vi "CLD 17 GUI number pad.vi"() -> ()   [LabVIEW 2015]
doc: "CLD 17\n\nThis VI uses a polling method to respond to changes in the GUI."
uses:
  CLD 17 Keypad_Typedef.ctl
panel:
  out "String":string="0"
  out "Numeric":dbl
  in  "Keypad Cluster":T1
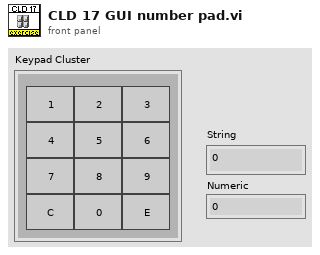
[diagram p1: front panel]
types:
  T1 = typedef "CLD 17 Keypad_Typedef.ctl" = cluster{"0":bool, "1":bool, "2":bool, "3":bool, "4":bool, "5":bool, "6":bool, "7":bool, "8":bool, "9":bool, "C":bool, "E":bool}
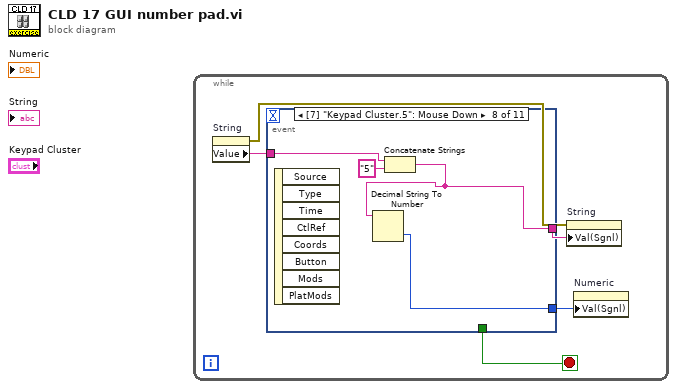
[diagram p0: block diagram]
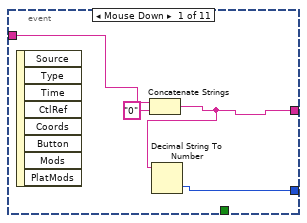
[diagram p2: hidden frame]
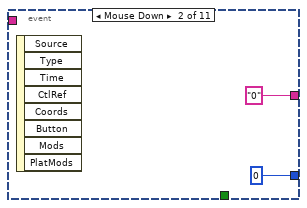
[diagram p3: hidden frame]
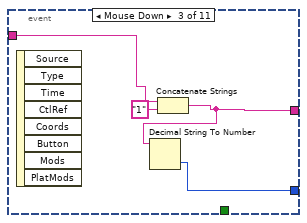
[diagram p4: hidden frame]
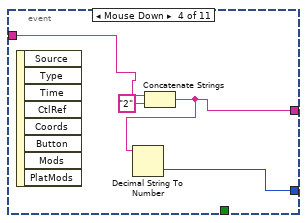
[diagram p5: hidden frame]
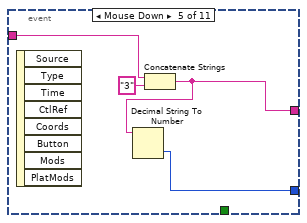
[diagram p6: hidden frame]
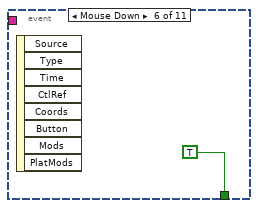
[diagram p7: hidden frame]
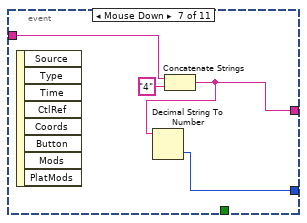
[diagram p8: hidden frame]
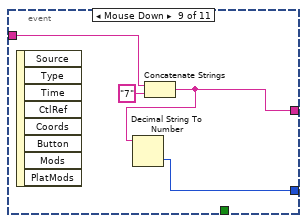
[diagram p9: hidden frame]
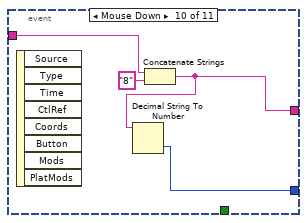
[diagram p10: hidden frame]
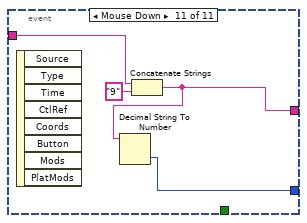
[diagram p11: hidden frame]
diagram:
  n1 = while {
    stop <- w5 stop-if-true
    n2 = property on="String" class="Str"() -> (error out=w2:errorcluster, "Value"=w4:string)  [unwired: 2 in, 1 out]
    n3 = event shown="[7] \"Keypad Cluster.5\": Mouse Down" {
      selector: _ -> [_ _ _ _ _ _ _ _ _ _ _]
      dyn-events: _ -> [_ _ _ _ _ _ _ _ _ _ _]
      timeout: _ -> [_ _ _ _ _ _ _ _ _ _ _]
      tunnel: [_ _ _ _ _ TRUE _ _ _ _ _] -> w5
      tunnel: w4 -> [w8 _ w14 w18 w22 _ w27 w30 w34 w37 w43]
      tunnel: [w6 "0" w12 w16 w21 _ w26 w31 w36 w39 w42] -> w3
      tunnel: [w7 0 w13 w17 w20 _ w25 w29 w33 w38 w41] -> w1
      event Mouse Down {
        n4 = event-data() -> ()  [unwired: 1 in, 8 out]
        n5 = Concatenate Strings(w8, "0" ("string")) -> (w6:string)
        n6 = Decimal String To Number(string=w6) -> (number=w7:i32)  [unwired: 2 in, 1 out]
      }
      event Mouse Down {
        n7 = event-data() -> ()  [unwired: 1 in, 8 out]
      }
      event Mouse Down {
        n8 = event-data() -> ()  [unwired: 1 in, 8 out]
        n9 = Concatenate Strings(w14, "1" ("string")) -> (w12:string)
        n10 = Decimal String To Number(string=w12) -> (number=w13:i32)  [unwired: 2 in, 1 out]
      }
      event Mouse Down {
        n11 = event-data() -> ()  [unwired: 1 in, 8 out]
        n12 = Concatenate Strings(w18, "2" ("string")) -> (w16:string)
        n13 = Decimal String To Number(string=w16) -> (number=w17:i32)  [unwired: 2 in, 1 out]
      }
      event Mouse Down {
        n14 = event-data() -> ()  [unwired: 1 in, 8 out]
        n15 = Concatenate Strings(w22, "3" ("string")) -> (w21:string)
        n16 = Decimal String To Number(string=w21) -> (number=w20:i32)  [unwired: 2 in, 1 out]
      }
      event Mouse Down {
        n17 = event-data() -> ()  [unwired: 1 in, 8 out]
      }
      event Mouse Down {
        n18 = event-data() -> ()  [unwired: 1 in, 8 out]
        n19 = Concatenate Strings(w27, "4" ("string")) -> (w26:string)
        n20 = Decimal String To Number(string=w26) -> (number=w25:i32)  [unwired: 2 in, 1 out]
      }
      event Mouse Down {
        n21 = event-data() -> ()  [unwired: 1 in, 8 out]
        n22 = Concatenate Strings(w30, "5" ("string")) -> (w31:string)
        n23 = Decimal String To Number(string=w31) -> (number=w29:i32)  [unwired: 2 in, 1 out]
      }
      event Mouse Down {
        n24 = event-data() -> ()  [unwired: 1 in, 8 out]
        n25 = Concatenate Strings(w34, "7" ("string")) -> (w36:string)
        n26 = Decimal String To Number(string=w36) -> (number=w33:i32)  [unwired: 2 in, 1 out]
      }
      event Mouse Down {
        n27 = event-data() -> ()  [unwired: 1 in, 8 out]
        n28 = Concatenate Strings(w37, "8" ("string")) -> (w39:string)
        n29 = Decimal String To Number(string=w39) -> (number=w38:i32)  [unwired: 2 in, 1 out]
      }
      event Mouse Down {
        n30 = event-data() -> ()  [unwired: 1 in, 8 out]
        n31 = Concatenate Strings(w43, "9" ("string")) -> (w42:string)
        n32 = Decimal String To Number(string=w42) -> (number=w41:i32)  [unwired: 2 in, 1 out]
      }
    }
    n33 = property on="String" class="Str"(error in=w2, "Val(Sgnl)"=w3) -> ()  [unwired: 1 in, 2 out]
    n34 = property on="Numeric" class="DigNum (strict)"("Val(Sgnl)"=w1) -> ()  [unwired: 2 in, 2 out]
  }
